vi "Continuous Serial Write and Read.vi"(8 "VISA resource name":refnum<visa-resource-name>="COM1", 9 "Read":bool, 10 "Write":bool, 11 "Command":string="*IDN?") -> (3 "Response":string)   [LabVIEW 2022 SP3]
doc: "This example performs writes and reads on a serial port, as directed by the user. You can press the Write and Read buttons, and change the Read Count, while the example is running.\n\nThe parameters set for the serial port must match the parameters of the connected instrument or device. In this example, the Read Count parameter specifies the number of bytes that the serial port reads. If there were more bytes at the port than the specified number, those bytes would not be read. If there were less bytes at the port than the specified number, you would receive a timeout error.\n\nThis example expands upon the flow control options for XON and XOFF, allowing the user to choose those control characters. Also, the user can enable or disable a termination character. Some devices require a termination character in order to identify the end of command strings. Some devices send a termination character to signify the end of data to be read. This example shows how you can end the Read operation once a termination character is detected in the buffer and/or append a termination character at the end of the Write data."
uses:
  Program Files (x86)/National Instruments/LabVIEW 2022/examples/Instrument IO/Serial/support/Serial - Settings.ctl
  Program Files (x86)/National Instruments/LabVIEW 2022/examples/Instrument IO/Serial/support/Serial - XON-XOFF Characters.ctl
  Program Files (x86)/National Instruments/LabVIEW 2022/examples/Instrument IO/Serial/support/Serial - ASCII Characters.ctl
  <vilib>/Instr/_visa.llb/VISA Configure Serial Port (Instr).vi
panel:
  in  "Termination Character":u8=10 format="%.0x"
  in  "Stop":bool
  in  "Read Count":u32=1000
  in  "XON/XOFF Characters":T1={"XON"=enum."DC1", "XOFF"=enum."DC3"}
  in  "Serial Settings":T3={"baud rate"=9600, "data bits"=8, "parity"=enum."None", "stop bits"=10, "flow control"=0} {"flow control" items=["None"=0, "XON/XOFF"=1, "RTS/CTS"=2, "DTR/DSR"=4]; "stop bits" items=["1.0"=10, "1.5"=15, "2.0"=20]; "data bits" min=5 max=8 step=1; "baud rate" items=["75"=75, "110"=110, "134"=134, "150"=150, "300"=300, "600"=600, "1200"=1200, "1800"=1800, "2400"=2400, "4800"=4800, "7200"=7200, "9600"=9600, "14400"=14400, "19200"=19200, "28800"=28800, "38400"=38400, "56000"=56000, "57600"=57600, "115200"=115200, "128000"=128000, "230400"=230400]}
  in  "End Read on Termination Character?":bool=TRUE
  # "Overview: Demonstrates the use of the VISA functions to write commands to and read responses from a serial instrument continuously in a loop.\nRequirements: NI-VISA Driver\nInstructions:\n1. Run the VI.\n2. Specify a Command and click the Write button.\n3. Read a Response by clicking the Read button.\n4. Click Stop to stop the VI."
  # "0xA is equivalent to a '\\n' character, which is a line feed."
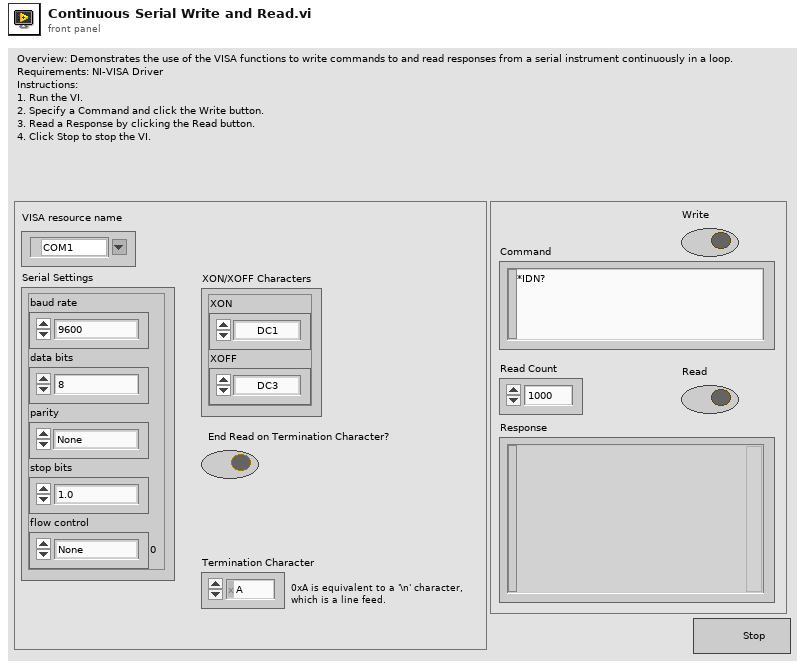
[diagram p1: front panel]
types:
  T1 = typedef "Serial - XON-XOFF Characters.ctl" = cluster{"XON":T2, "XOFF":T2}
  T2 = typedef "Serial - ASCII Characters.ctl" = enum16{"NUL", "SOH", "STX", "ETX", "EOT", "ENQ", "ACK", "BEL", "BS", "HT", "LF", "VT", "FF", "CR", "SO", "SI", "DLE", "DC1", "DC2", "DC3", "DC4", "NAK", "SYN", "ETB", "CAN", "EM", "SUB", "ESC", "FS", "GS", "RS", "US", "SP", "!", "\"", "#", "$", "%", "&", "'", "(", ")", "*", "+", ",", "- (-)", ".", "/", "0", "1", "2", "3", "4", "5", "6", "7", "8", "9", ":", ";", "<", "=", ">", "?", "@", "A", "B", "C", "D", "E", "F", "G", "H", "I", "J", "K", "L", "M", "N", "O", "P", "Q", "R", "S", "T", "U", "V", "W", "X", "Y", "Z", "[", "\\", "]", "^", "_", "`", "a", "b", "c", "d", "e", "f", "g", "h", "i", "j", "k", "l", "m", "n", "o", "p", "q", "r", "s", "t", "u", "v", "w", "x", "y", "z", "{", "|", "}", "~"}
  T3 = typedef "Serial - Settings.ctl" = cluster{"baud rate":u32, "data bits":u16, "parity":enum16{"None", "Odd", "Even", "Mark", "Space"}, "stop bits":u16, "flow control":u16}
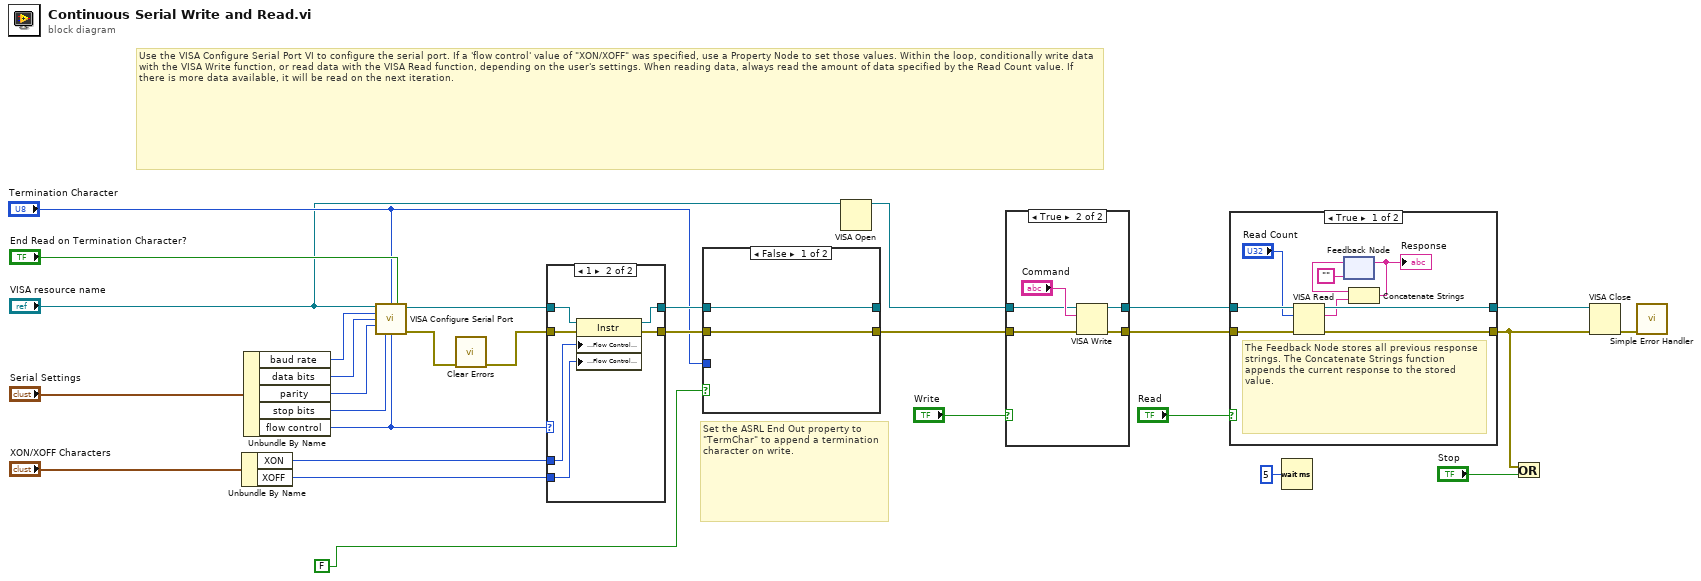
[diagram p0: block diagram]
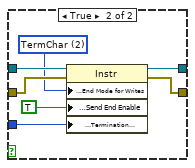
[diagram p4: hidden frame]
diagram:
  # "Set the ASRL End Out property to \"TermChar\" to append a termination character on write."
  # "Use the VISA Configure Serial Port VI to configure the serial port. If a 'flow control' value of \"XON/XOFF\" was specified, use a Property Node to set those values. Within the loop, conditionally write data with the VISA Write function, or read data with the VISA Read function, depending on the user's settings. When reading data, always read the amount of data specified by the Read Count value. If there is more data available, it will be read on the next iteration."
  n1 = Unbundle By Name("XON/XOFF Characters") -> ("XON"=w16:T2, "XOFF"=w15:T2)
  n2 = Unbundle By Name("Serial Settings") -> ("baud rate"=w23:u32, "data bits"=w24:u16, "parity"=w25:enum16{"None", "Odd", "Even", "Mark", "Space"}, "stop bits"=w26:u16, "flow control"=w17:u16)
  n3 = call-poly "VISA Configure Serial Port"("VISA resource name"="VISA resource name", "termination char\n(0xA = '\\n' = LF)"="Termination Character", "Enable Termination\nChar (T)"="End Read on Termination Character?", "baud rate (9600)"=w23, "data bits (8)"=w24, "parity (0:none)"=w25, "stop bits (10: 1 bit)"=w26, "flow control (0:none)"=w17) -> ("VISA resource name out"=w27:refnum<visa-resource-name>, "error out"=w28:errorcluster)  [unwired: 2 in, 4 out]
  n4 = call <vilib>:"Clear Errors.vi"("error in (no error)"=w28) -> ("error out"=w10:errorcluster)  [unwired: 5 in, 1 out]
  n5 = case shown="1" w17 {
    tunnel: [w30 w37] -> w14
    tunnel: [w31 w36] -> w12
    tunnel: w10 -> [w30 w35]
    tunnel: w27 -> [w31 w34]
    tunnel: w16 -> [_ w33]
    tunnel: w15 -> [_ w32]
    frame Default {
    }
    frame 1 {
      n6 = property class="Instr"(reference=w34, error in=w35, "Serial Settings:Flow Control XON Character"=w33, "Serial Settings:Flow Control XOFF Character"=w32) -> (reference out=w36:refnum<visa-resource-name>, error out=w37:errorcluster)
    }
  }
  n7 = case shown="False" FALSE {
    tunnel: w12 -> [w38 w46]
    tunnel: w14 -> [w39 w45]
    tunnel: [w38 w44] -> _
    tunnel: [w39 w43] -> w13
    tunnel: "Termination Character" -> [_ w41]
    frame False {
    }
    frame True {
      w42 = u16 2 items=["None", "LastBit", "TermChar", "Break"] ("Serial Settings:Serial End Mode for Writes")
      n8 = property class="Instr"(reference=w46, error in=w45, "Serial Settings:End Mode for Writes"=w42, "Message Based Settings:Send End Enable"=TRUE, "Message Based Settings:Termination Character"=w41) -> (reference out=w44:refnum<visa-resource-name>, error out=w43:errorcluster)
    }
  }
  n9 = VISA Open(VISA resource name="VISA resource name") -> (VISA resource name=w8:refnum<visa-resource-name>)  [unwired: 4 in, 1 out]
  n10 = case shown="True" "Write" {
    tunnel: w8 -> [w48 w52]
    tunnel: w13 -> [w47 w51]
    tunnel: [w48 w50] -> w7
    tunnel: [w47 w49] -> w6
    frame False {
    }
    frame True {
      n11 = VISA Write(VISA resource name=w52, write buffer="Command", error in (no error)=w51) -> (VISA resource name out=w50:refnum<visa-resource-name>, error out=w49:errorcluster)  [unwired: 1 out]
    }
  }
  n12 = case shown="True" "Read" {
    tunnel: [w60 w64] -> w18
    tunnel: w7 -> [w62 w64]
    tunnel: [w58 w63] -> w19
    tunnel: w6 -> [w61 w63]
    frame True {
      # "The Feedback Node stores all previous response strings. The Concatenate Strings function appends the current response to the stored value."
      n13 = VISA Read(VISA resource name=w62, byte count="Read Count", error in (no error)=w61) -> (VISA resource name out=w60:refnum<visa-resource-name>, read buffer=w57:string, error out=w58:errorcluster)  [unwired: 1 out]
      n14 = feedback #1("") -> (w56:string)
      n15 = Concatenate Strings(w56, w57) -> (w55:string)
      "Response" <- w55
      n16 = feedback-in #1(w55) -> ()
    }
    frame False {
    }
  }
  n17 = Wait (ms)(milliseconds to wait=u32 5) -> ()  [unwired: 1 out]
  n18 = Or(x=w19, y="Stop") -> ()  [unwired: 1 out]
  n19 = VISA Close(VISA resource name=w18, error in (no error)=w19) -> (error out=w20:errorcluster)
  n20 = call <vilib>:"Simple Error Handler.vi"("error in (no error)"=w20) -> ()  [unwired: 1 in, 8 out]
